vi "LED patterns.vi"() -> ()   [LabVIEW 2023]
uses:
  ctrl defs/ctrl number of LEDs.ctl
  ctrl defs/ctrl LED PATTERN DEFS.ctl
  ctrl defs/ctrl LED PATTERN SHAPES.ctl
  <vilib>/Rock Robotics/WPI/ThirdParty/JAS_Junk/TrajLib/MathUtil_Clamp.vi
  <vilib>/Rock Robotics/WPI/ThirdParty/JAS_Junk/TrajLib/Util_GetTime.vi
  <vilib>/Rock Robotics/WPI/ThirdParty/JAS_Junk/TrajLib/VI/Util_GetTime_U32.vi
  Global odometry.vi
  <vilib>/Rock Robotics/SystemInterfaces/Utilities/FPGA_UtilitiesRead LocalTime.vi
  <vilib>/Rock Robotics/WPI/ThirdParty/JAS_Junk/TrajLib/VI/Util_GetTime_U64.vi
  Global INIT.vi
  <vilib>/Rock Robotics/WPI/ThirdParty/JAS_Junk/TrajLib/Trajectory_Library.lvlib
panel:
  out "PATTERN SELECTED":T1=enum."WHITE, PULSE"
  out "decimated array 2":dbl[](array[numeric])
  out "decimated array":dbl[](array[numeric])
  out "Numeric":dbl
  out "FIBONACCI array":dbl[](array[numeric])
  out "HEARTBEAT":i32=54716
  in  "Dk BLUE":u32(colorbox)=721055
  in  "FUSCIA":u32(colorbox)=13107455
  in  "VIOLET":u32(colorbox)=5249480
  in  "PINK":u32(colorbox)=16070299
  in  "YELLOW":u32(colorbox)=16776960
  in  "ORANGE":u32(colorbox)=15156737
  in  "GREEN":u32(colorbox)=65280
  in  "Color2":u32(colorbox)=14535680 caption="Team\nColor\nSECOND"
  in  "Color1":u32(colorbox)=20922 caption="Team\nColor\nMAIN"
  out "SINE 0-1":dbl=0.9567727288213003
  out "SCAN rotation":dbl=47.83863644106501
  out "array DK BLUE":u32[](array[numeric])=[721055, 721055, 721055, 721055, 721055, 721055, 721055, 721055, 721055, 721055, 721055, 721055, 721055, 721055, 721055, 721055, 721055, 721055, 721055, 721055, 721055, 721055, 721055, 721055, 721055, 721055, 721055, 721055, 721055, 721055, 721055, 721055, 721055, 721055, 721055, 721055, 721055, 721055, 721055, 721055, 721055, 721055, 721055, 721055, 721055, 721055, 721055, 721055, 721055, 721055, 721055, 721055, 721055, 721055, 721055, 721055, 721055, 721055, 721055, 721055]
  in  "TESTING?":bool
  out "error out":errorcluster
  in  "error in (no error)":errorcluster
  out "LED WRITE 3":u32[](array[colorbox])
  out "LED WRITE 2":u32[](array[colorbox])=[0, 0, 0, 0, 0, 0, 0, 0, 20922, 20922, 20922, 20922, 20922, 20922, 20922, 20922, 20922, 20922, 0, 0]
  out "LED WRITE":u32[](array[colorbox])=[0, 0, 14535680, 14535680, 14535680, 14535680, 14535680, 14535680, 14535680, 14535680, 14535680, 14535680, 0, 0, 0, 0, 0, 0, 0, 0, 0, 0, 0, 0, 0, 0, 0, 0, 0, 0, 0, 0, 0, 0, 0, 0, 0, 0, 0, 0, 0, 0, 0, 0, 0, 0, 0, 0, 20922, 20922, 20922, 20922, 20922, 20922, 20922, 20922, 20922, 20922, 0, 0]
  in  "LOOP - BLINK (ms)":dbl=25.0
  in  "LOOP - BUMPER (ms)":dbl=10.0
  in  "LOOP - SCAN (ms)":dbl=10.0
  in  "LOOP - PULSE (ms)":dbl=10.0
  in  "LOOP - WAVE (ms)":dbl=10.0
  out "AdjustedWaitTime_MS":u32
  in  "DesiredLoopTime_MS":dbl=25.0 format="%#_13g"
  out "array AQUA":u32[](array[numeric])=[61414, 61414, 61414, 61414, 61414, 61414, 61414, 61414, 61414, 61414, 61414, 61414, 61414, 61414, 61414, 61414, 61414, 61414, 61414, 61414, 61414, 61414, 61414, 61414, 61414, 61414, 61414, 61414, 61414, 61414, 61414, 61414, 61414, 61414, 61414, 61414, 61414, 61414, 61414, 61414, 61414, 61414, 61414, 61414, 61414, 61414, 61414, 61414, 61414, 61414, 61414, 61414, 61414, 61414, 61414, 61414, 61414, 61414, 61414, 61414]
  out "array PINK":u32[](array[numeric])=[16711808, 16711808, 16711808, 16711808, 16711808, 16711808, 16711808, 16711808, 16711808, 16711808, 16711808, 16711808, 16711808, 16711808, 16711808, 16711808, 16711808, 16711808, 16711808, 16711808, 16711808, 16711808, 16711808, 16711808, 16711808, 16711808, 16711808, 16711808, 16711808, 16711808, 16711808, 16711808, 16711808, 16711808, 16711808, 16711808, 16711808, 16711808, 16711808, 16711808, 16711808, 16711808, 16711808, 16711808, 16711808, 16711808, 16711808, 16711808, 16711808, 16711808, 16711808, 16711808, 16711808, 16711808, 16711808, 16711808, 16711808, 16711808, 16711808, 16711808]
  out "array YELLOW":u32[](array[numeric])=[16449369, 16449369, 16449369, 16449369, 16449369, 16449369, 16449369, 16449369, 16449369, 16449369, 16449369, 16449369, 16449369, 16449369, 16449369, 16449369, 16449369, 16449369, 16449369, 16449369, 16449369, 16449369, 16449369, 16449369, 16449369, 16449369, 16449369, 16449369, 16449369, 16449369, 16449369, 16449369, 16449369, 16449369, 16449369, 16449369, 16449369, 16449369, 16449369, 16449369, 16449369, 16449369, 16449369, 16449369, 16449369, 16449369, 16449369, 16449369, 16449369, 16449369, 16449369, 16449369, 16449369, 16449369, 16449369, 16449369, 16449369, 16449369, 16449369, 16449369]
  out "SINE WAVE 1/2":u32[](array[numeric])=[0, 3, 11, 24, 42, 64, 88, 114, 141, 167, 191, 213, 231, 244, 252, 255, 252, 244, 231, 213, 191, 167, 141, 114, 88, 64, 42, 24, 11, 3, 0, 3, 11, 24, 42, 64, 88, 114, 141, 167, 191, 213, 231, 244, 252, 255, 252, 244, 231, 213, 191, 167, 141, 114, 88, 64, 42, 24, 11, 3]
  out "SINE WAVE":u32[](array[numeric])=[0, 1, 3, 6, 11, 17, 24, 33, 42, 53, 64, 76, 88, 101, 114, 128, 141, 154, 167, 179, 191, 202, 213, 222, 231, 238, 244, 249, 252, 254, 255, 254, 252, 249, 244, 238, 231, 222, 213, 202, 191, 179, 167, 154, 141, 128, 114, 101, 88, 76, 64, 53, 42, 33, 24, 17, 11, 6, 3, 1]
  out "REVERSE BUMP":i8=49
  out "FORWARD INDEX":i32=29
  out "REVERSE INDEX":i32=30
  in  "slider length":i8=10
  out "array EMPTY":u32[](array[numeric])=[1073741824, 1073741824, 1073741824, 1073741824, 1073741824, 1073741824, 1073741824, 1073741824, 1073741824, 1073741824, 1073741824, 1073741824, 1073741824, 1073741824, 1073741824, 1073741824, 1073741824, 1073741824, 1073741824, 1073741824, 1073741824, 1073741824, 1073741824, 1073741824, 1073741824, 1073741824, 1073741824, 1073741824, 1073741824, 1073741824, 1073741824, 1073741824, 1073741824, 1073741824, 1073741824, 1073741824, 1073741824, 1073741824, 1073741824, 1073741824, 1073741824, 1073741824, 1073741824, 1073741824, 1073741824, 1073741824, 1073741824, 1073741824, 1073741824, 1073741824, 1073741824, 1073741824, 1073741824, 1073741824, 1073741824, 1073741824, 1073741824, 1073741824, 1073741824, 1073741824]
  out "SLIDER BLACK":u32[](array[colorbox])
  out "array BLUE":u32[](array[numeric])=[220, 220, 220, 220, 220, 220, 220, 220, 220, 220, 220, 220, 220, 220, 220, 220, 220, 220, 220, 220, 220, 220, 220, 220, 220, 220, 220, 220, 220, 220, 220, 220, 220, 220, 220, 220, 220, 220, 220, 220, 220, 220, 220, 220, 220, 220, 220, 220, 220, 220, 220, 220, 220, 220, 220, 220, 220, 220, 220, 220]
  out "array FUSCIA":u32[](array[numeric])=[16711934, 16711934, 16711934, 16711934, 16711934, 16711934, 16711934, 16711934, 16711934, 16711934, 16711934, 16711934, 16711934, 16711934, 16711934, 16711934, 16711934, 16711934, 16711934, 16711934, 16711934, 16711934, 16711934, 16711934, 16711934, 16711934, 16711934, 16711934, 16711934, 16711934, 16711934, 16711934, 16711934, 16711934, 16711934, 16711934, 16711934, 16711934, 16711934, 16711934, 16711934, 16711934, 16711934, 16711934, 16711934, 16711934, 16711934, 16711934, 16711934, 16711934, 16711934, 16711934, 16711934, 16711934, 16711934, 16711934, 16711934, 16711934, 16711934, 16711934]
  out "array ORANGE":u32[](array[numeric])=[16748288, 16748288, 16748288, 16748288, 16748288, 16748288, 16748288, 16748288, 16748288, 16748288, 16748288, 16748288, 16748288, 16748288, 16748288, 16748288, 16748288, 16748288, 16748288, 16748288, 16748288, 16748288, 16748288, 16748288, 16748288, 16748288, 16748288, 16748288, 16748288, 16748288, 16748288, 16748288, 16748288, 16748288, 16748288, 16748288, 16748288, 16748288, 16748288, 16748288, 16748288, 16748288, 16748288, 16748288, 16748288, 16748288, 16748288, 16748288, 16748288, 16748288, 16748288, 16748288, 16748288, 16748288, 16748288, 16748288, 16748288, 16748288, 16748288, 16748288]
  out "array COLOR1":u32[](array[numeric])=[191, 191, 191, 191, 191, 191, 191, 191, 191, 191, 191, 191, 191, 191, 191, 191, 191, 191, 191, 191, 191, 191, 191, 191, 191, 191, 191, 191, 191, 191, 191, 191, 191, 191, 191, 191, 191, 191, 191, 191, 191, 191, 191, 191, 191, 191, 191, 191, 191, 191, 191, 191, 191, 191, 191, 191, 191, 191, 191, 191]
  out "array COLOR2":u32[](array[numeric])=[14794496, 14794496, 14794496, 14794496, 14794496, 14794496, 14794496, 14794496, 14794496, 14794496, 14794496, 14794496, 14794496, 14794496, 14794496, 14794496, 14794496, 14794496, 14794496, 14794496, 14794496, 14794496, 14794496, 14794496, 14794496, 14794496, 14794496, 14794496, 14794496, 14794496, 14794496, 14794496, 14794496, 14794496, 14794496, 14794496, 14794496, 14794496, 14794496, 14794496, 14794496, 14794496, 14794496, 14794496, 14794496, 14794496, 14794496, 14794496, 14794496, 14794496, 14794496, 14794496, 14794496, 14794496, 14794496, 14794496, 14794496, 14794496, 14794496, 14794496]
  out "array RED":u32[](array[numeric])=[16711680, 16711680, 16711680, 16711680, 16711680, 16711680, 16711680, 16711680, 16711680, 16711680, 16711680, 16711680, 16711680, 16711680, 16711680, 16711680, 16711680, 16711680, 16711680, 16711680, 16711680, 16711680, 16711680, 16711680, 16711680, 16711680, 16711680, 16711680, 16711680, 16711680, 16711680, 16711680, 16711680, 16711680, 16711680, 16711680, 16711680, 16711680, 16711680, 16711680, 16711680, 16711680, 16711680, 16711680, 16711680, 16711680, 16711680, 16711680, 16711680, 16711680, 16711680, 16711680, 16711680, 16711680, 16711680, 16711680, 16711680, 16711680, 16711680, 16711680]
  out "array GREEN":u32[](array[numeric])=[65280, 65280, 65280, 65280, 65280, 65280, 65280, 65280, 65280, 65280, 65280, 65280, 65280, 65280, 65280, 65280, 65280, 65280, 65280, 65280, 65280, 65280, 65280, 65280, 65280, 65280, 65280, 65280, 65280, 65280, 65280, 65280, 65280, 65280, 65280, 65280, 65280, 65280, 65280, 65280, 65280, 65280, 65280, 65280, 65280, 65280, 65280, 65280, 65280, 65280, 65280, 65280, 65280, 65280, 65280, 65280, 65280, 65280, 65280, 65280]
  out "array WHITE":u32[](array[numeric])=[16448250, 16448250, 16448250, 16448250, 16448250, 16448250, 16448250, 16448250, 16448250, 16448250, 16448250, 16448250, 16448250, 16448250, 16448250, 16448250, 16448250, 16448250, 16448250, 16448250, 16448250, 16448250, 16448250, 16448250, 16448250, 16448250, 16448250, 16448250, 16448250, 16448250, 16448250, 16448250, 16448250, 16448250, 16448250, 16448250, 16448250, 16448250, 16448250, 16448250, 16448250, 16448250, 16448250, 16448250, 16448250, 16448250, 16448250, 16448250, 16448250, 16448250, 16448250, 16448250, 16448250, 16448250, 16448250, 16448250, 16448250, 16448250, 16448250, 16448250]
  out "array BLACK":u32[](array[numeric])
  out "array VIOLET":u32[](array[numeric])=[11152127, 11152127, 11152127, 11152127, 11152127, 11152127, 11152127, 11152127, 11152127, 11152127, 11152127, 11152127, 11152127, 11152127, 11152127, 11152127, 11152127, 11152127, 11152127, 11152127, 11152127, 11152127, 11152127, 11152127, 11152127, 11152127, 11152127, 11152127, 11152127, 11152127, 11152127, 11152127, 11152127, 11152127, 11152127, 11152127, 11152127, 11152127, 11152127, 11152127, 11152127, 11152127, 11152127, 11152127, 11152127, 11152127, 11152127, 11152127, 11152127, 11152127, 11152127, 11152127, 11152127, 11152127, 11152127, 11152127, 11152127, 11152127, 11152127, 11152127]
  out "SLIDER WHITE":u32[](array[colorbox])=[16448250, 16448250, 16448250, 16448250, 16448250, 16448250, 16448250, 16448250, 16448250, 16448250]
  in  "TEST - PATTERN SELECT":T1=enum."CROSSING, COLORS 1&2"
  out "#LEDs":T2=60
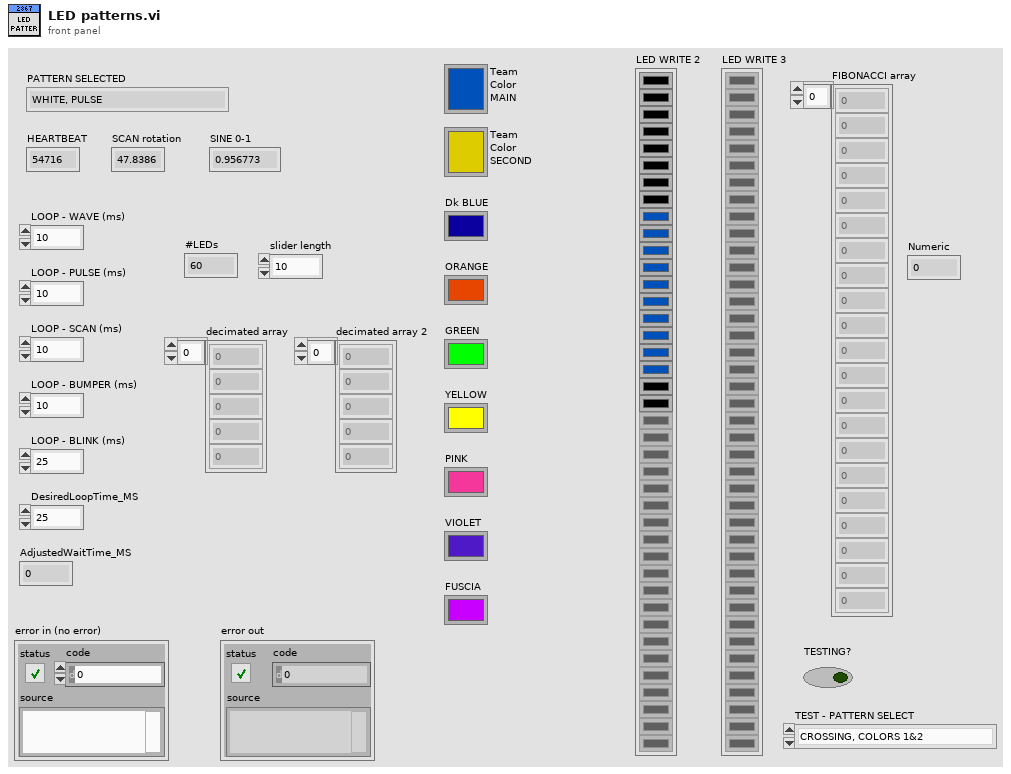
[diagram p1: front panel]
types:
  T1 = typedef "ctrl LED PATTERN DEFS.ctl" = enum16{"default", "RED, SOLID", "RED, BUMPER", "RED, BLINK", "RED, WAVE", "RED, SCAN", "RED, PULSE", "BLUE, SOLID", "BLUE, BUMPER", "BLUE, BLINK", "BLUE, WAVE", "BLUE, SCAN", "BLUE, PULSE", "GREEN, SOLID", "GREEN, BUMPER", "GREEN, BLINK", "GREEN, WAVE", "GREEN, SCAN", "GREEN, PULSE", "WHITE, WAVE", "WHITE, PULSE", "COLOR 1 scan white", "COLOR 1 scan COLOR 2", "COLOR 1 bumper white", "COLOR 1 bumper COLOR 2", "PINK, SOLID", "PINK, BLINK", "VIOLET, SOLID", "VIOLET, BLINK", "ORANGE, SOLID", "ORANGE, BLINK", "YELLOW, SOLID", "YELLOW, BLINK", "FUSCIA, SOLID", "FUSCIA, BLINK", "AQUA, SOLID", "AQUA, BLINK", "AQUA, BUMPER", "AQUA, SCAN", "FUSCIA, BUMPER", "FUSCIA, SCAN", "ORANGE, BUMPER", "ORANGE, SCAN", "VIOLET, BUMPER", "VIOLET, SCAN", "YELLOW, BUMPER", "YELLOW, SCAN", "PINK, BUMPER", "PINK, SCAN", "CROSSING, RED & BLUE", "CROSSING, COLORS 1&2", "TEST", "RAINBOW", "RED, EXPAND", "BLUE, EXPAND", "GREEN, EXPAND", "RED, EX-CON", "BLUE, EX-CON", "GREEN, EX-CON", "EMERGENCY STOP", "LOW BATTERY"}
  T2 = typedef "ctrl number of LEDs.ctl" = u16
  T3 = typedef "ctrl LED PATTERN SHAPES.ctl" = enum16{"SOLID", "BUMPER", "SCAN", "WAVE", "EXPAND", "EX-CON", "CROSS", "BLINK", "PULSE", "SCAN FAST", "BUMPER FAST", "FIBONACCI"}
  T4 = typedef "ctrl LED init.ctl" = cluster{"PWM Channel":T5, "refnum name":string, "#LEDS":T2, "initial output":dbl, "stack name":string, "Installed?":bool, "pattern":T6}
  T5 = typedef "FPGA_DIOPWMChannel.ctl" = enum8{"PWM 0", "PWM 1", "PWM 2", "PWM 3", "PWM 4", "PWM 5", "PWM 6", "PWM 7", "PWM 8", "PWM 9", "PWM MXP 0", "PWM MXP 1", "PWM MXP 2", "PWM MXP 3", "PWM MXP 4", "PWM MXP 5", "PWM MXP 6", "PWM MXP 7", "PWM MXP 8", "PWM MXP 9", "Invalid"}
  T6 = typedef "ctrl LED PATTERNS.ctl" = u16
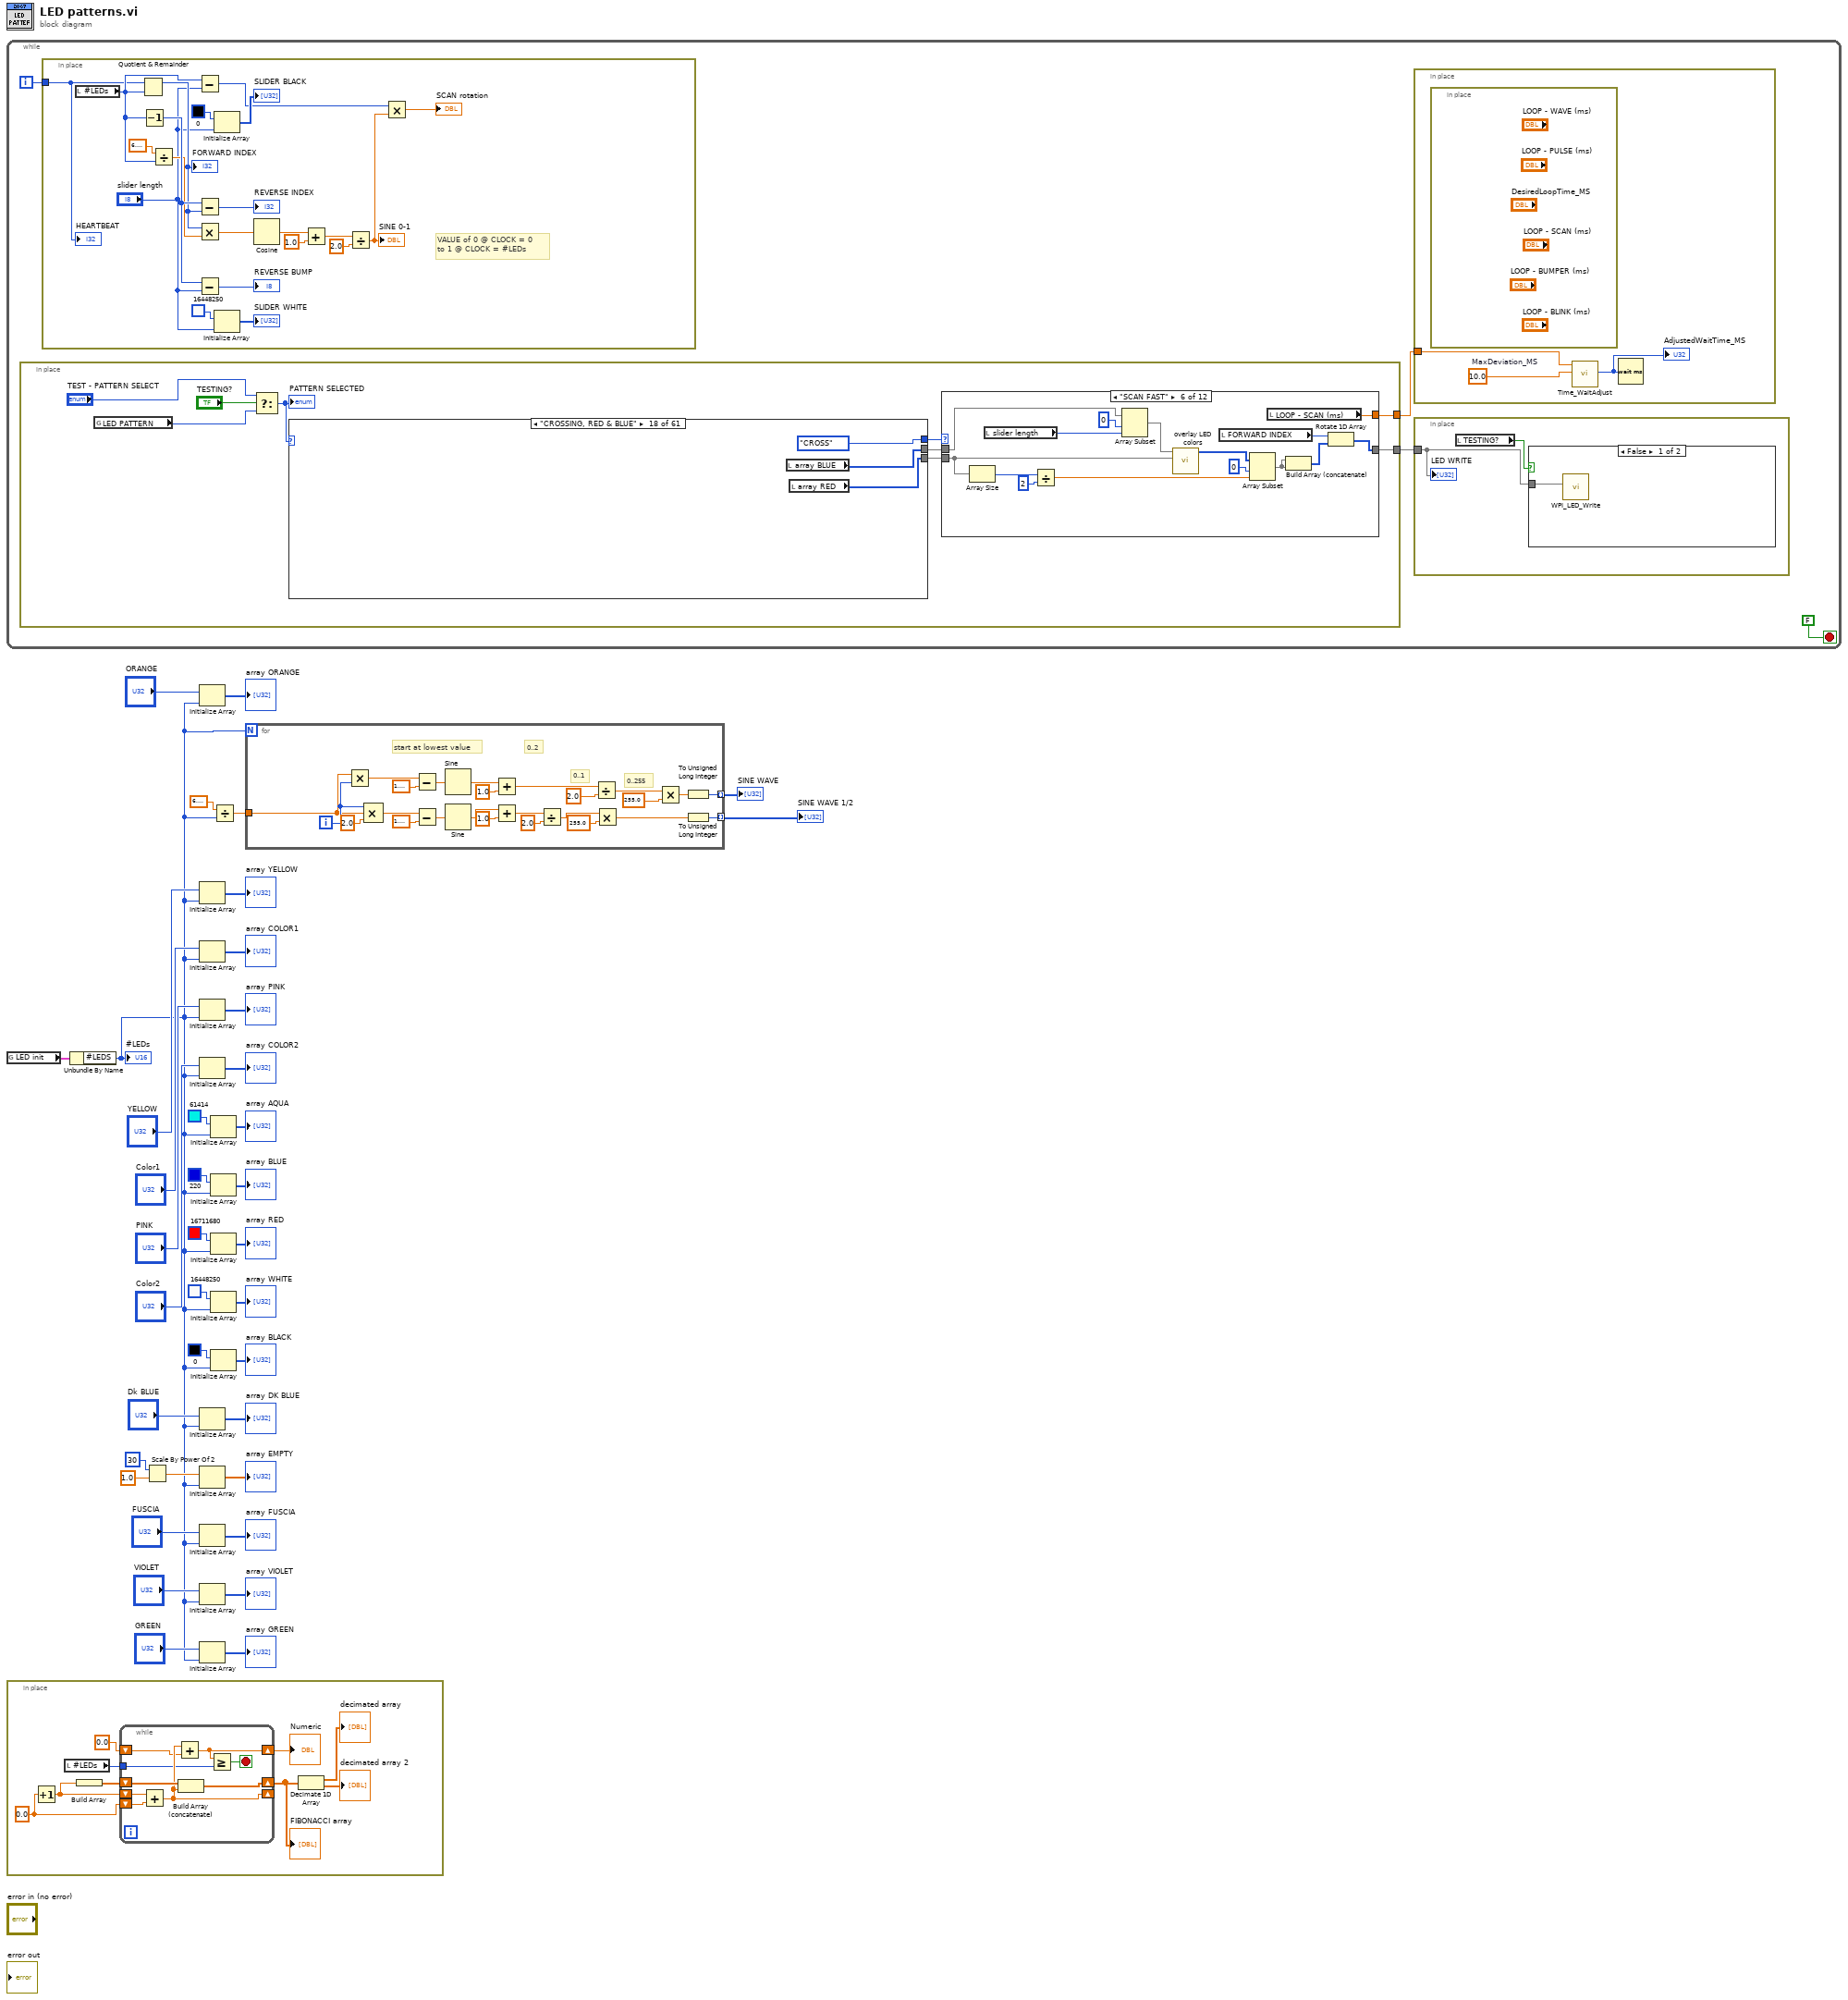
[diagram p0: block diagram]
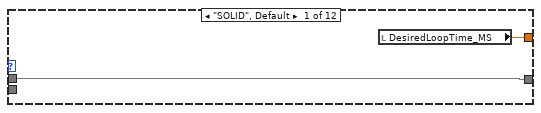
[diagram p2: hidden frame]
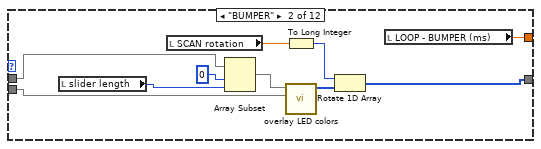
[diagram p3: hidden frame]
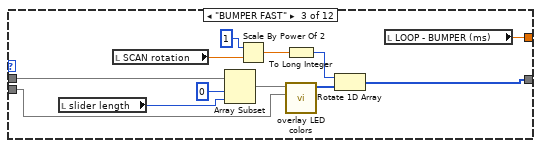
[diagram p4: hidden frame]
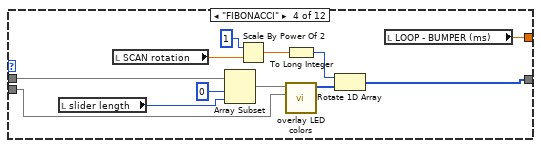
[diagram p5: hidden frame]
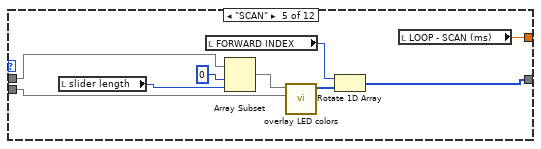
[diagram p6: hidden frame]
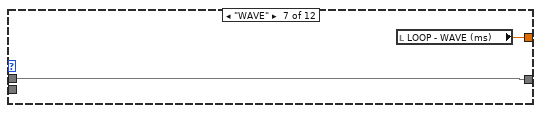
[diagram p7: hidden frame]
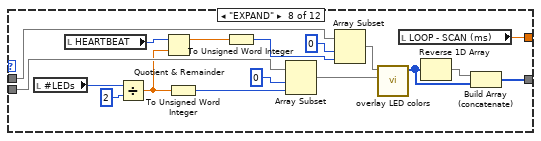
[diagram p8: hidden frame]
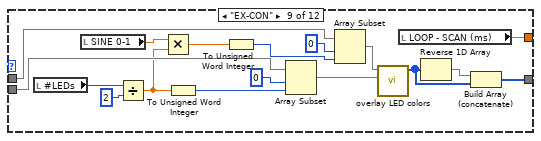
[diagram p9: hidden frame]
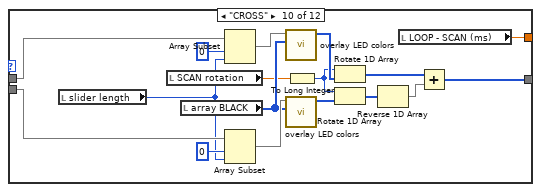
[diagram p10: hidden frame]
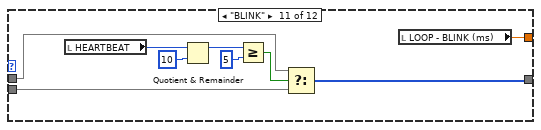
[diagram p11: hidden frame]
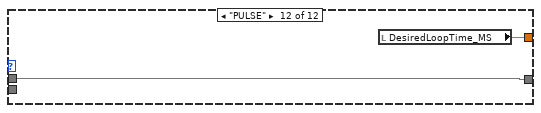
[diagram p12: hidden frame]
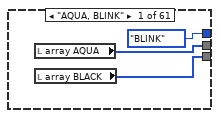
[diagram p13: hidden frame]
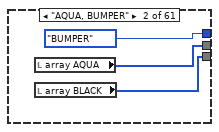
[diagram p14: hidden frame]
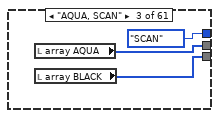
[diagram p15: hidden frame]
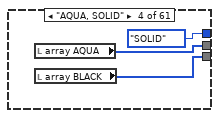
[diagram p16: hidden frame]
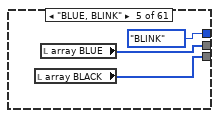
[diagram p17: hidden frame]
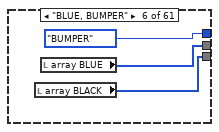
[diagram p18: hidden frame]
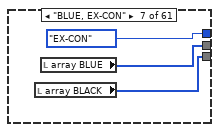
[diagram p19: hidden frame]
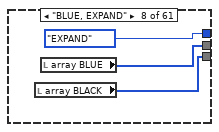
[diagram p20: hidden frame]
diagram:
  n1 = while {
    i -> [w42]
    stop <- FALSE stop-if-true
    n2 = in-place {
      in-place-border: [w50] -> w41
      in-place-border: [w48] -> w40
      n3 = global read "Global odometry.vi" "LED PATTERN"() -> (w43:T1)
      n4 = Select(t="TEST - PATTERN SELECT", s="TESTING?", f=w43) -> (s? t:f=w46:T1)
      "PATTERN SELECTED" <- w46
      n5 = case shown="\"CROSSING, RED & BLUE\"" w46 {
        tunnel: [w178 w181 w184 w187 w190 w193 w196 w199 w206 w209 w211 w218 w221 w223 w226 w240 w246 w249 w252 w256 w259 w262 w265 w268 w271 w274 w277 w284 w287 w290 w297 w300 w303 w306 w309 w311 w315 w318 w321 w323 w335 w337 w341 w344 w351 w354 w356 w363 w366 w369 w372 w377 w390 w410 w412 w414 w425 w437 w440 w443 w446] -> w51
        tunnel: [w177 w180 w183 w186 w189 w192 w195 w198 w201 w208 w211 w213 w220 w224 w226 w240 w247 w250 w252 w255 w258 w261 w264 w267 w270 w273 w276 w279 w286 w289 w292 w299 w302 w305 w308 w310 w314 w317 w320 w323 w334 w338 w340 w343 w346 w353 w356 w358 w365 w368 w371 w377 w390 w409 w411 w414 w425 w436 w439 w442 w445] -> w49
        tunnel: [ctrl_LED_PATTERN_SHAPES."BLINK" ctrl_LED_PATTERN_SHAPES."BUMPER" ctrl_LED_PATTERN_SHAPES."SCAN" ctrl_LED_PATTERN_SHAPES."SOLID" ctrl_LED_PATTERN_SHAPES."BLINK" ctrl_LED_PATTERN_SHAPES."BUMPER" ctrl_LED_PATTERN_SHAPES."EX-CON" ctrl_LED_PATTERN_SHAPES."EXPAND" ctrl_LED_PATTERN_SHAPES."PULSE" ctrl_LED_PATTERN_SHAPES."SCAN" ctrl_LED_PATTERN_SHAPES."SOLID" ctrl_LED_PATTERN_SHAPES."WAVE" ctrl_LED_PATTERN_SHAPES."BUMPER" ctrl_LED_PATTERN_SHAPES."BUMPER" ctrl_LED_PATTERN_SHAPES."SOLID" ctrl_LED_PATTERN_SHAPES."SCAN" ctrl_LED_PATTERN_SHAPES."CROSS" ctrl_LED_PATTERN_SHAPES."CROSS" ctrl_LED_PATTERN_SHAPES."SOLID" ctrl_LED_PATTERN_SHAPES."BLINK" ctrl_LED_PATTERN_SHAPES."BUMPER" ctrl_LED_PATTERN_SHAPES."SCAN" ctrl_LED_PATTERN_SHAPES."SOLID" ctrl_LED_PATTERN_SHAPES."BLINK" ctrl_LED_PATTERN_SHAPES."BUMPER" ctrl_LED_PATTERN_SHAPES."EX-CON" ctrl_LED_PATTERN_SHAPES."EXPAND" ctrl_LED_PATTERN_SHAPES."PULSE" ctrl_LED_PATTERN_SHAPES."SCAN" ctrl_LED_PATTERN_SHAPES."SOLID" ctrl_LED_PATTERN_SHAPES."WAVE" ctrl_LED_PATTERN_SHAPES."BLINK" ctrl_LED_PATTERN_SHAPES."BUMPER" ctrl_LED_PATTERN_SHAPES."SCAN FAST" ctrl_LED_PATTERN_SHAPES."SOLID" ctrl_LED_PATTERN_SHAPES."BLINK" ctrl_LED_PATTERN_SHAPES."BUMPER" ctrl_LED_PATTERN_SHAPES."SCAN" ctrl_LED_PATTERN_SHAPES."SOLID" ctrl_LED_PATTERN_SHAPES."SOLID" ctrl_LED_PATTERN_SHAPES."BLINK" ctrl_LED_PATTERN_SHAPES."BUMPER" ctrl_LED_PATTERN_SHAPES."EX-CON" ctrl_LED_PATTERN_SHAPES."EXPAND" ctrl_LED_PATTERN_SHAPES."PULSE" ctrl_LED_PATTERN_SHAPES."SCAN FAST" ctrl_LED_PATTERN_SHAPES."SOLID" ctrl_LED_PATTERN_SHAPES."WAVE" ctrl_LED_PATTERN_SHAPES."SCAN" ctrl_LED_PATTERN_SHAPES."BLINK" ctrl_LED_PATTERN_SHAPES."BUMPER" ctrl_LED_PATTERN_SHAPES."SCAN" ctrl_LED_PATTERN_SHAPES."SCAN" ctrl_LED_PATTERN_SHAPES."SCAN" ctrl_LED_PATTERN_SHAPES."SOLID" ctrl_LED_PATTERN_SHAPES."SOLID" ctrl_LED_PATTERN_SHAPES."SOLID" ctrl_LED_PATTERN_SHAPES."BLINK" ctrl_LED_PATTERN_SHAPES."BUMPER" ctrl_LED_PATTERN_SHAPES."SCAN" ctrl_LED_PATTERN_SHAPES."SOLID"] -> w47
        frame "AQUA, BLINK" {
          n6 = local read "array AQUA"() -> (w178:u32[])
          n7 = local read "array BLACK"() -> (w177:u32[])
        }
        frame "AQUA, BUMPER" {
          n8 = local read "array AQUA"() -> (w181:u32[])
          n9 = local read "array BLACK"() -> (w180:u32[])
        }
        frame "AQUA, SCAN" {
          n10 = local read "array AQUA"() -> (w184:u32[])
          n11 = local read "array BLACK"() -> (w183:u32[])
        }
        frame "AQUA, SOLID" {
          n12 = local read "array AQUA"() -> (w187:u32[])
          n13 = local read "array BLACK"() -> (w186:u32[])
        }
        frame "BLUE, BLINK" {
          n14 = local read "array BLACK"() -> (w189:u32[])
          n15 = local read "array BLUE"() -> (w190:u32[])
        }
        frame "BLUE, BUMPER" {
          n16 = local read "array BLACK"() -> (w192:u32[])
          n17 = local read "array BLUE"() -> (w193:u32[])
        }
        frame "BLUE, EX-CON" {
          n18 = local read "array BLACK"() -> (w195:u32[])
          n19 = local read "array BLUE"() -> (w196:u32[])
        }
        frame "BLUE, EXPAND" {
          n20 = local read "array BLACK"() -> (w198:u32[])
          n21 = local read "array BLUE"() -> (w199:u32[])
        }
        frame "BLUE, PULSE" {
          n22 = local read "SINE WAVE 1/2"() -> (w205:u32[])
          n23 = local read "FORWARD INDEX"() -> (w204:i32)
          n24 = Logical Shift(y=i16 0, x=w205) -> (x << y=w203:u32[])
          n25 = local read "array BLACK"() -> (w201:u32[])
          n26 = Rotate 1D Array(1:w203, 2:w204) -> (0:w206:u32[])
        }
        frame "BLUE, SCAN" {
          n27 = local read "array BLACK"() -> (w208:u32[])
          n28 = local read "array BLUE"() -> (w209:u32[])
        }
        frame "BLUE, SOLID" {
          n29 = local read "array BLUE"() -> (w211:u32[])
        }
        frame "BLUE, WAVE" {
          n30 = local read "SINE WAVE"() -> (w217:u32[])
          n31 = local read "FORWARD INDEX"() -> (w216:i32)
          n32 = Logical Shift(y=i16 0, x=w217) -> (x << y=w215:u32[])
          n33 = local read "array BLACK"() -> (w213:u32[])
          n34 = Rotate 1D Array(1:w215, 2:w216) -> (0:w218:u32[])
        }
        frame "COLOR 1 bumper COLOR 2" {
          n35 = local read "array COLOR2"() -> (w221:u32[])
          n36 = local read "array COLOR1"() -> (w220:u32[])
        }
        frame "COLOR 1 bumper white" {
          n37 = local read "array COLOR1"() -> (w224:u32[])
          n38 = local read "array WHITE"() -> (w223:u32[])
        }
        frame "COLOR 1 scan COLOR 2" {
          n39 = local read "Color2"() -> (w236:u32)
          n40 = Initialize Array(w236, 10 ("dimension size")) -> (w235:u32[])
          n41 = local read "array COLOR1"() -> (w238:u32[])
          n42 = local read "#LEDs"() -> (w231:T2)
          n43 = call "overlay LED colors.vi"("BASE ARRAY"=w238, "OVERLAY"=w235) -> ("BLENDED ARRAY"=w233:u32[])  [unwired: 9 in]
          n44 = Quotient & Remainder(x=w231, y=i8 3) -> (floor(x/y)=w229:T2)  [unwired: 1 out]
          n45 = local read "FORWARD INDEX"() -> (w237:i32)
          n46 = Array Subset(array=w233, index=0, length=w229) -> (w228:u32[])
          n47 = Build Array (concatenate)(w228, w228, w228) -> (w227:u32[])
          n48 = Rotate 1D Array(1:w227, 2:w237) -> (0:w226:u32[])
        }
        frame "COLOR 1 scan white" {
          n49 = local read "SLIDER WHITE"() -> (w244:u32[])
          n50 = local read "array COLOR1"() -> (w243:u32[])
          n51 = local read "FORWARD INDEX"() -> (w241:i32)
          n52 = call "overlay LED colors.vi"("BASE ARRAY"=w243, "OVERLAY"=w244) -> ("BLENDED ARRAY"=w242:u32[])  [unwired: 9 in]
          n53 = Rotate 1D Array(1:w242, 2:w241) -> (0:w240:u32[])
        }
        frame "CROSSING, COLORS 1&2" {
          n54 = local read "array COLOR1"() -> (w246:u32[])
          n55 = local read "array COLOR2"() -> (w247:u32[])
        }
        frame "CROSSING, RED & BLUE" {
          n56 = local read "array BLUE"() -> (w249:u32[])
          n57 = local read "array RED"() -> (w250:u32[])
        }
        frame "default", Default {
          n58 = local write "TEST - PATTERN SELECT"(ctrl_LED_PATTERN_DEFS."COLOR 1 bumper COLOR 2" ("PATTERN SELECT")) -> ()
          n59 = local read "array BLACK"() -> (w252:u32[])
        }
        frame "FUSCIA, BLINK" {
          n60 = local read "array FUSCIA"() -> (w256:u32[])
          n61 = local read "array BLACK"() -> (w255:u32[])
        }
        frame "FUSCIA, BUMPER" {
          n62 = local read "array FUSCIA"() -> (w259:u32[])
          n63 = local read "array BLACK"() -> (w258:u32[])
        }
        frame "FUSCIA, SCAN" {
          n64 = local read "array FUSCIA"() -> (w262:u32[])
          n65 = local read "array BLACK"() -> (w261:u32[])
        }
        frame "FUSCIA, SOLID" {
          n66 = local read "array FUSCIA"() -> (w265:u32[])
          n67 = local read "array BLACK"() -> (w264:u32[])
        }
        frame "GREEN, BLINK" {
          n68 = local read "array GREEN"() -> (w268:u32[])
          n69 = local read "array BLACK"() -> (w267:u32[])
        }
        frame "GREEN, BUMPER" {
          n70 = local read "array GREEN"() -> (w271:u32[])
          n71 = local read "array BLACK"() -> (w270:u32[])
        }
        frame "GREEN, EX-CON" {
          n72 = local read "array GREEN"() -> (w274:u32[])
          n73 = local read "array BLACK"() -> (w273:u32[])
        }
        frame "GREEN, EXPAND" {
          n74 = local read "array GREEN"() -> (w277:u32[])
          n75 = local read "array BLACK"() -> (w276:u32[])
        }
        frame "GREEN, PULSE" {
          n76 = local read "SINE WAVE 1/2"() -> (w283:u32[])
          n77 = local read "FORWARD INDEX"() -> (w282:i32)
          n78 = Logical Shift(y=i16 8, x=w283) -> (x << y=w281:u32[])
          n79 = local read "array BLACK"() -> (w279:u32[])
          n80 = Rotate 1D Array(1:w281, 2:w282) -> (0:w284:u32[])
        }
        frame "GREEN, SCAN" {
          n81 = local read "array GREEN"() -> (w287:u32[])
          n82 = local read "array BLACK"() -> (w286:u32[])
        }
        frame "GREEN, SOLID" {
          n83 = local read "array GREEN"() -> (w290:u32[])
          n84 = local read "array BLACK"() -> (w289:u32[])
        }
        frame "GREEN, WAVE" {
          n85 = local read "SINE WAVE"() -> (w296:u32[])
          n86 = local read "FORWARD INDEX"() -> (w295:i32)
          n87 = Logical Shift(y=i16 8, x=w296) -> (x << y=w294:u32[])
          n88 = local read "array BLACK"() -> (w292:u32[])
          n89 = Rotate 1D Array(1:w294, 2:w295) -> (0:w297:u32[])
        }
        frame "ORANGE, BLINK" {
          n90 = local read "array ORANGE"() -> (w300:u32[])
          n91 = local read "array BLACK"() -> (w299:u32[])
        }
        frame "ORANGE, BUMPER" {
          n92 = local read "array ORANGE"() -> (w303:u32[])
          n93 = local read "array BLACK"() -> (w302:u32[])
        }
        frame "ORANGE, SCAN" {
          n94 = local read "array ORANGE"() -> (w306:u32[])
          n95 = local read "array BLACK"() -> (w305:u32[])
        }
        frame "ORANGE, SOLID" {
          n96 = local read "array ORANGE"() -> (w309:u32[])
          n97 = local read "array BLACK"() -> (w308:u32[])
        }
        frame "PINK, BLINK" {
          n98 = local read "array BLACK"() -> (w310:u32[])
          n99 = local read "array PINK"() -> (w311:u32[])
        }
        frame "PINK, BUMPER" {
          n100 = local read "array BLACK"() -> (w314:u32[])
          n101 = local read "array PINK"() -> (w315:u32[])
        }
        frame "PINK, SCAN" {
          n102 = local read "array BLACK"() -> (w317:u32[])
          n103 = local read "array PINK"() -> (w318:u32[])
        }
        frame "PINK, SOLID" {
          n104 = local read "array BLACK"() -> (w320:u32[])
          n105 = local read "array PINK"() -> (w321:u32[])
        }
        frame "RAINBOW" {
          n106 = local read "SINE WAVE"() -> (w328:u32[])
          n107 = local read "FORWARD INDEX"() -> (w326:i32)
          n108 = Logical Shift(y=i16 0, x=w328) -> (x << y=w331:u32[])
          n109 = Logical Shift(y=i16 16, x=w328) -> (x << y=w327:u32[])
          n110 = Rotate 1D Array(1:w331, 2:w326) -> (0:w332:u32[])
          n111 = Rotate 1D Array(1:w327, 2:w326) -> (0:w325:u32[])
          n112 = Reverse 1D Array(array=w325) -> (reversed array=w324:u32[])
          n113 = Add(x=w332, y=w324) -> (x+y=w323:u32[])
        }
        frame "RED, BLINK" {
          n114 = local read "array BLACK"() -> (w334:u32[])
          n115 = local read "array RED"() -> (w335:u32[])
        }
        frame "RED, BUMPER" {
          n116 = local read "array BLACK"() -> (w338:u32[])
          n117 = local read "array RED"() -> (w337:u32[])
        }
        frame "RED, EX-CON" {
          n118 = local read "array BLACK"() -> (w340:u32[])
          n119 = local read "array RED"() -> (w341:u32[])
        }
        frame "RED, EXPAND" {
          n120 = local read "array BLACK"() -> (w343:u32[])
          n121 = local read "array RED"() -> (w344:u32[])
        }
        frame "RED, PULSE" {
          n122 = local read "SINE WAVE 1/2"() -> (w350:u32[])
          n123 = local read "FORWARD INDEX"() -> (w349:i32)
          n124 = Logical Shift(y=i16 16, x=w350) -> (x << y=w348:u32[])
          n125 = local read "array BLACK"() -> (w346:u32[])
          n126 = Rotate 1D Array(1:w348, 2:w349) -> (0:w351:u32[])
        }
        frame "RED, SCAN" {
          n127 = local read "array BLACK"() -> (w353:u32[])
          n128 = local read "array RED"() -> (w354:u32[])
        }
        frame "RED, SOLID" {
          n129 = local read "array RED"() -> (w356:u32[])
        }
        frame "RED, WAVE" {
          n130 = local read "SINE WAVE"() -> (w362:u32[])
          n131 = local read "FORWARD INDEX"() -> (w361:i32)
          n132 = Logical Shift(y=i16 16, x=w362) -> (x << y=w360:u32[])
          n133 = local read "array BLACK"() -> (w358:u32[])
          n134 = Rotate 1D Array(1:w360, 2:w361) -> (0:w363:u32[])
        }
        frame "TEST" {
          n135 = local read "array BLACK"() -> (w365:u32[])
          n136 = local read "array PINK"() -> (w366:u32[])
        }
        frame "VIOLET, BLINK" {
          n137 = local read "array VIOLET"() -> (w369:u32[])
          n138 = local read "array BLACK"() -> (w368:u32[])
        }
        frame "VIOLET, BUMPER" {
          n139 = local read "array VIOLET"() -> (w372:u32[])
          n140 = local read "array BLACK"() -> (w371:u32[])
        }
        frame "EMERGENCY STOP" {
          w382 = 0 ("index")
          n141 = local read "#LEDs"() -> (w385:T2)
          n142 = local read "array YELLOW"() -> (w383:u32[])
          n143 = local read "array RED"() -> (w375:u32[])
          n144 = Quotient & Remainder(x=w385, y=T2 8) -> (x-y*floor(x/y)=w373:T2, floor(x/y)=w381:T2)
          n145 = Array Subset(array=w375, index=w382, length=w381) -> (w380:u32[])
          n146 = Array Subset(array=w383, index=w382, length=w381) -> (w379:u32[])
          n147 = Array Subset(array=w375, index=0, length=w373) -> (w376:u32[])
          n148 = Build Array (concatenate)(w380, w379) -> (w378:u32[])
          n149 = Build Array (concatenate)(w378, w378, w378, w378, w376) -> (w377:u32[])
        }
        frame "LOW BATTERY" {
          w403 = 0 ("index")
          w401 = T2 3 ("y")
          n150 = local read "array YELLOW"() -> (w402:u32[])
          n151 = local read "array RED"() -> (w397:u32[])
          n152 = local read "#LEDs"() -> (w388:T2)
          n153 = Array Subset(array=w397, index=w403, length=w401) -> (w400:u32[])
          n154 = Array Subset(array=w402, index=w403, length=w401) -> (w399:u32[])
          n155 = Quotient & Remainder(x=w388, y=w401) -> (x-y*floor(x/y)=w395:T2, floor(x/y)=w398:T2)
          n156 = Build Array (concatenate)(w400, w399) -> (w391:u32[])
          n157 = for {
            N: w398 -> [_]
            tunnel: w391 -> [w406]
            shift-right: [w405] -> w394
            shift-left: w391 -> [w407]
            n158 = Build Array (concatenate)(w407, w406) -> (w405:u32[])
          }
          n159 = Array Subset(array=w397, index=0, length=w395) -> (w393:u32[])
          n160 = Build Array (concatenate)(w394, w393) -> (w392:u32[])
          n161 = Decrement(x=w388) -> (x-1=w387:T2)
          n162 = Array Subset(array=w392, index=0, length=w387) -> (w390:u32[])
        }
        frame "VIOLET, SCAN" {
          n163 = local read "array VIOLET"() -> (w410:u32[])
          n164 = local read "array BLACK"() -> (w409:u32[])
        }
        frame "VIOLET, SOLID" {
          n165 = local read "array VIOLET"() -> (w412:u32[])
          n166 = local read "array BLACK"() -> (w411:u32[])
        }
        frame "WHITE, PULSE" {
          n167 = local read "SINE WAVE 1/2"() -> (w416:u32[])
          n168 = local read "FORWARD INDEX"() -> (w424:i32)
          n169 = Logical Shift(y=i16 0, x=w416) -> (x << y=w419:u32[])
          n170 = Logical Shift(y=i16 8, x=w416) -> (x << y=w418:u32[])
          n171 = Logical Shift(y=i16 16, x=w416) -> (x << y=w417:u32[])
          n172 = Compound Arithmetic op=ADD(w419, w418, w417) -> (w420:u32[])
          n173 = Rotate 1D Array(1:w420, 2:w424) -> (0:w414:u32[])
        }
        frame "WHITE, WAVE" {
          n174 = local read "SINE WAVE"() -> (w427:u32[])
          n175 = local read "FORWARD INDEX"() -> (w435:i32)
          n176 = Logical Shift(y=i16 0, x=w427) -> (x << y=w430:u32[])
          n177 = Logical Shift(y=i16 8, x=w427) -> (x << y=w429:u32[])
          n178 = Logical Shift(y=i16 16, x=w427) -> (x << y=w428:u32[])
          n179 = Compound Arithmetic op=ADD(w430, w429, w428) -> (w431:u32[])
          n180 = Rotate 1D Array(1:w431, 2:w435) -> (0:w425:u32[])
        }
        frame "YELLOW, BLINK" {
          n181 = local read "array YELLOW"() -> (w437:u32[])
          n182 = local read "array BLACK"() -> (w436:u32[])
        }
        frame "YELLOW, BUMPER" {
          n183 = local read "array YELLOW"() -> (w440:u32[])
          n184 = local read "array BLACK"() -> (w439:u32[])
        }
        frame "YELLOW, SCAN" {
          n185 = local read "array YELLOW"() -> (w443:u32[])
          n186 = local read "array BLACK"() -> (w442:u32[])
        }
        frame "YELLOW, SOLID" {
          n187 = local read "array YELLOW"() -> (w446:u32[])
          n188 = local read "array BLACK"() -> (w445:u32[])
        }
      }
      n189 = case shown="\"SCAN FAST\"" w47 {
        tunnel: w51 -> [w53 w59 w71 w83 w94 w109 w113 w123 w140 w161 w169 w175]
        tunnel: [w53 w56 w68 w80 w91 w106 w113 w127 w144 w163 w167 w175] -> w50
        tunnel: w49 -> [_ w55 w67 w79 w90 w102 _ w122 w139 w160 w168 _]
        tunnel: [w52 w54 w66 w78 w88 w104 w112 w114 w131 w148 w165 w174] -> w48
        frame "SOLID", Default {
          n190 = local read "DesiredLoopTime_MS"() -> (w52:dbl)
        }
        frame "BUMPER" {
          n191 = local read "slider length"() -> (w57:i8)
          n192 = local read "SCAN rotation"() -> (w62:dbl)
          n193 = Array Subset(array=w59, index=0, length=w57) -> (w60:u32[])
          n194 = To Long Integer(number=w62) -> (32bit integer=w61:i32)
          n195 = call "overlay LED colors.vi"("BASE ARRAY"=w55, "OVERLAY"=w60) -> ("BLENDED ARRAY"=w63:u32[])  [unwired: 9 in]
          n196 = Rotate 1D Array(1:w63, 2:w61) -> (0:w56:u32[])
          n197 = local read "LOOP - BUMPER (ms)"() -> (w54:dbl)
        }
        frame "BUMPER FAST" {
          n198 = local read "slider length"() -> (w69:i8)
          n199 = local read "SCAN rotation"() -> (w74:dbl)
          n200 = Array Subset(array=w71, index=0, length=w69) -> (w72:u32[])
          n201 = Scale By Power Of 2(n=i16 1, x=w74) -> (x*2^n=w65:dbl)
          n202 = To Long Integer(number=w65) -> (32bit integer=w73:i32)
          n203 = call "overlay LED colors.vi"("BASE ARRAY"=w67, "OVERLAY"=w72) -> ("BLENDED ARRAY"=w75:u32[])  [unwired: 9 in]
          n204 = Rotate 1D Array(1:w75, 2:w73) -> (0:w68:u32[])
          n205 = local read "LOOP - BUMPER (ms)"() -> (w66:dbl)
        }
        frame "FIBONACCI" {
          n206 = local read "slider length"() -> (w81:i8)
          n207 = local read "SCAN rotation"() -> (w86:dbl)
          n208 = Array Subset(array=w83, index=0, length=w81) -> (w84:u32[])
          n209 = Scale By Power Of 2(n=i16 1, x=w86) -> (x*2^n=w77:dbl)
          n210 = To Long Integer(number=w77) -> (32bit integer=w85:i32)
          n211 = call "overlay LED colors.vi"("BASE ARRAY"=w79, "OVERLAY"=w84) -> ("BLENDED ARRAY"=w87:u32[])  [unwired: 9 in]
          n212 = Rotate 1D Array(1:w87, 2:w85) -> (0:w80:u32[])
          n213 = local read "LOOP - BUMPER (ms)"() -> (w78:dbl)
        }
        frame "SCAN" {
          n214 = local read "slider length"() -> (w92:i8)
          n215 = local read "FORWARD INDEX"() -> (w89:i32)
          n216 = Array Subset(array=w94, index=0, length=w92) -> (w95:u32[])
          n217 = call "overlay LED colors.vi"("BASE ARRAY"=w90, "OVERLAY"=w95) -> ("BLENDED ARRAY"=w96:u32[])  [unwired: 9 in]
          n218 = Rotate 1D Array(1:w96, 2:w89) -> (0:w91:u32[])
          n219 = local read "LOOP - SCAN (ms)"() -> (w88:dbl)
        }
        frame "SCAN FAST" {
          n220 = Array Size(array=w102) -> (size(s)=w100:i32)
          n221 = local read "slider length"() -> (w107:i8)
          n222 = Divide(x=w100, y=2) -> (x/y=w101:dbl)
          n223 = Array Subset(array=w109, index=0, length=w107) -> (w110:u32[])
          n224 = call "overlay LED colors.vi"("BASE ARRAY"=w102, "OVERLAY"=w110) -> ("BLENDED ARRAY"=w111:u32[])  [unwired: 9 in]
          n225 = local read "FORWARD INDEX"() -> (w105:i32)
          n226 = Array Subset(array=w111, index=0, length=w101) -> (w97:u32[])
          n227 = local read "LOOP - SCAN (ms)"() -> (w104:dbl)
          n228 = Build Array (concatenate)(w97, w97) -> (w98:u32[])
          n229 = Rotate 1D Array(1:w98, 2:w105) -> (0:w106:u32[])
        }
        frame "WAVE" {
          n230 = local read "LOOP - WAVE (ms)"() -> (w112:dbl)
        }
        frame "EXPAND" {
          n231 = local read "#LEDs"() -> (w118:T2)
          n232 = local read "HEARTBEAT"() -> (w115:i32)
          n233 = Divide(x=w118, y=u16 2) -> (x/y=w120:dbl)
          n234 = Quotient & Remainder(x=w115, y=w120) -> (x-y*floor(x/y)=w119:dbl)  [unwired: 1 out]
          n235 = To Unsigned Word Integer(number=w120) -> (unsigned 16bit integer=w117:u16)
          n236 = To Unsigned Word Integer(number=w119) -> (unsigned 16bit integer=w116:u16)
          n237 = Array Subset(array=w122, index=0, length=w117) -> (w124:u32[])
          n238 = Array Subset(array=w123, index=0, length=w116) -> (w130:u32[])
          n239 = call "overlay LED colors.vi"("BASE ARRAY"=w124, "OVERLAY"=w130) -> ("BLENDED ARRAY"=w126:u32[])  [unwired: 9 in]
          n240 = local read "LOOP - SCAN (ms)"() -> (w114:dbl)
          n241 = Reverse 1D Array(array=w126) -> (reversed array=w128:u32[])
          n242 = Build Array (concatenate)(w128, w126) -> (w127:u32[])
        }
        frame "EX-CON" {
          n243 = local read "#LEDs"() -> (w135:T2)
          n244 = local read "SINE 0-1"() -> (w132:dbl)
          n245 = Divide(x=w135, y=u16 2) -> (x/y=w137:dbl)
          n246 = Multiply(x=w132, y=w137) -> (x*y=w136:dbl)
          n247 = To Unsigned Word Integer(number=w137) -> (unsigned 16bit integer=w134:u16)
          n248 = To Unsigned Word Integer(number=w136) -> (unsigned 16bit integer=w133:u16)
          n249 = Array Subset(array=w139, index=0, length=w134) -> (w141:u32[])
          n250 = Array Subset(array=w140, index=0, length=w133) -> (w147:u32[])
          n251 = call "overlay LED colors.vi"("BASE ARRAY"=w141, "OVERLAY"=w147) -> ("BLENDED ARRAY"=w143:u32[])  [unwired: 9 in]
          n252 = local read "LOOP - SCAN (ms)"() -> (w131:dbl)
          n253 = Reverse 1D Array(array=w143) -> (reversed array=w145:u32[])
          n254 = Build Array (concatenate)(w145, w143) -> (w144:u32[])
        }
        frame "CROSS" {
          n255 = local read "slider length"() -> (w159:i8)
          n256 = local read "SCAN rotation"() -> (w153:dbl)
          n257 = local read "array BLACK"() -> (w156:u32[])
          n258 = Array Subset(array=w161, index=0, length=w159) -> (w157:u32[])
          n259 = Array Subset(array=w160, index=0, length=w159) -> (w158:u32[])
          n260 = call "overlay LED colors.vi"("BASE ARRAY"=w156, "OVERLAY"=w157) -> ("BLENDED ARRAY"=w155:u32[])  [unwired: 9 in]
          n261 = call "overlay LED colors.vi"("BASE ARRAY"=w156, "OVERLAY"=w158) -> ("BLENDED ARRAY"=w154:u32[])  [unwired: 9 in]
          n262 = To Long Integer(number=w153) -> (32bit integer=w152:i32)
          n263 = Rotate 1D Array(1:w155, 2:w152) -> (0:w151:u32[])
          n264 = Rotate 1D Array(1:w154, 2:w152) -> (0:w150:u32[])
          n265 = Reverse 1D Array(array=w150) -> (reversed array=w149:u32[])
          n266 = local read "LOOP - SCAN (ms)"() -> (w148:dbl)
          n267 = Add(x=w151, y=w149) -> (x+y=w163:u32[])
        }
        frame "BLINK" {
          n268 = local read "HEARTBEAT"() -> (w166:i32)
          n269 = Quotient & Remainder(x=w166, y=10) -> (x-y*floor(x/y)=w172:i32)  [unwired: 1 out]
          n270 = Greater Or Equal?(x=w172, y=5) -> (x >= y?=w170:bool)
          n271 = Select(t=w169, s=w170, f=w168) -> (s? t:f=w167:u32[])
          n272 = local read "LOOP - BLINK (ms)"() -> (w165:dbl)
        }
        frame "PULSE" {
          n273 = local read "DesiredLoopTime_MS"() -> (w174:dbl)
        }
      }
    }
    n274 = in-place {
      in-place-border: w42 -> [w449]
      # "VALUE of 0 @ CLOCK = 0\nto 1 @ CLOCK = #LEDs"
      n275 = local read "#LEDs"() -> (w453:T2)
      n276 = Quotient & Remainder(x=w449, y=w453) -> (x-y*floor(x/y)=w459:i32)  [unwired: 1 out]
      "FORWARD INDEX" <- w459
      n277 = Decrement(x=w453) -> (x-1=w462:T2)
      n278 = Divide(x=6.283185307179586, y=w453) -> (x/y=w460:dbl)
      n279 = Subtract(x=w453, y="slider length") -> (x-y=w451:T2)
      n280 = Subtract(x=w462, y=w459) -> (x-y=→"REVERSE INDEX":i32)
      n281 = Multiply(x=w459, y=w460) -> (x*y=w458:dbl)
      n282 = Subtract(x=w462, y="slider length") -> (x-y=→"REVERSE BUMP":T2)
      n283 = Initialize Array(u32 0 ("Color2"), "slider length") -> (→"SLIDER BLACK":u32[])
      n284 = Initialize Array(u32 16448250 ("Color2"), "slider length") -> (→"SLIDER WHITE":u32[])
      n285 = Cosine(x=w458) -> (cos(x)=w457:dbl)
      n286 = Add(x=w457, y=1.0) -> (x+y=w455:dbl)
      n287 = Divide(x=w455, y=2.0) -> (x/y=w448:dbl)
      "SINE 0-1" <- w448
      n288 = Multiply(x=w451, y=w448) -> (x*y=→"SCAN rotation":dbl)
      "HEARTBEAT" <- w449
    }
    n289 = in-place {
      in-place-border: w40 -> [w469]
      w471 = 10.0  # MaxDeviation_MS
      n290 = in-place {
      }
      n291 = call <vilib>:"Time_WaitAdjust.vi"("MaxAdjustment_MS"=w471, "DesiredLoopTime_MS"=w469) -> ("AdjustedWaitTime_MS"=w470:u32)  [unwired: 8 in, 1 out]
      "AdjustedWaitTime_MS" <- w470
      n292 = Wait (ms)(milliseconds to wait=w470) -> ()  [unwired: 1 out]
    }
    n293 = in-place {
      in-place-border: w41 -> [w472]
      n294 = local read "TESTING?"() -> (w473:bool)
      n295 = case shown="False" w473 {
        tunnel: w472 -> [w474 w476]
        frame False {
          n296 = call <vilib>:"WPI_LED_Write.vi"("Color Array"=w474) -> ()  [unwired: 10 in, 1 out]
        }
        frame True {
          n297 = local read "#LEDs"() -> (w478:T2)
          n298 = Divide(x=w478, y=T2 2) -> (x/y=w475:dbl)
          n299 = Split 1D Array(array=w476, index=w475) -> (first subarray=→"LED WRITE 2":u32[], second subarray=→"LED WRITE 3":u32[])
        }
      }
      "LED WRITE" <- w472
    }
  }
  n300 = global read "Global INIT.vi" "LED init"() -> (w2:T4)
  n301 = in-place {
    w488 = 0.0 ("element")
    n302 = Increment(x=w488) -> (x+1=w487:dbl)
    n303 = local read "#LEDs"() -> (w484:T2)
    n304 = Build Array(w487) -> (w489:dbl[])
    n305 = while {
      shift-right: [w494] -> _
      shift-left: w487 -> [w496]
      shift-left: w488 -> [w495]
      shift-right: [w497] -> w483
      shift-left: w489 -> [w498]
      shift-right: [w491] -> w485
      shift-left: 0.0 -> [w493]
      tunnel: w484 -> [w490]
      stop <- w492 stop-if-true
      n306 = Add(x=w496, y=w495) -> (x+y=w494:dbl)
      n307 = Add(x=w494, y=w493) -> (x+y=w491:dbl)
      n308 = Build Array (concatenate)(w498, w494) -> (w497:dbl[])
      n309 = Greater Or Equal?(x=w491, y=w490) -> (x >= y?=w492:bool)
    }
    "FIBONACCI array" <- w483
    "Numeric" <- w485
    n310 = Decimate 1D Array(w483) -> (→"decimated array":dbl[], →"decimated array 2":dbl[])
  }
  n311 = Unbundle By Name(w2) -> ("#LEDS"=w1:T2)
  "#LEDs" <- w1
  n312 = Scale By Power Of 2(n=i16 30, x=1.0) -> (x*2^n=w19:dbl)
  n313 = Initialize Array("ORANGE", w1) -> (→"array ORANGE":u32[])
  n314 = Initialize Array("YELLOW", w1) -> (→"array YELLOW":u32[])
  n315 = Initialize Array("Color1", w1) -> (→"array COLOR1":u32[])
  n316 = Initialize Array("PINK", w1) -> (→"array PINK":u32[])
  n317 = Initialize Array("Color2", w1) -> (→"array COLOR2":u32[])
  n318 = Initialize Array("Dk BLUE", w1) -> (→"array DK BLUE":u32[])
  n319 = Initialize Array(w19, w1) -> (→"array EMPTY":dbl[])
  n320 = Initialize Array("FUSCIA", w1) -> (→"array FUSCIA":u32[])
  n321 = Initialize Array("VIOLET", w1) -> (→"array VIOLET":u32[])
  n322 = Initialize Array("GREEN", w1) -> (→"array GREEN":u32[])
  n323 = Initialize Array(u32 61414 ("Color2"), w1) -> (→"array AQUA":u32[])
  n324 = Initialize Array(u32 220 ("Color2"), w1) -> (→"array BLUE":u32[])
  n325 = Initialize Array(u32 16711680 ("Color2"), w1) -> (→"array RED":u32[])
  n326 = Initialize Array(u32 16448250 ("Color2"), w1) -> (→"array WHITE":u32[])
  n327 = Initialize Array(u32 0 ("Color2"), w1) -> (→"array BLACK":u32[])
  n328 = Divide(x=6.283185307179586, y=w1) -> (x/y=w13:dbl)
  n329 = for {
    N: w1 -> [_]
    tunnel: w13 -> [w502]
    tunnel: [w514] -> w12 mode=indexing
    tunnel: [w500] -> w11 mode=indexing
    i -> [w503]
    # "0..255"
    # "start at lowest value"
    # "0..1"
    # "0..2"
    n330 = Multiply(x=w502, y=w503) -> (x*y=w519:dbl)
    n331 = Compound Arithmetic op=MULTIPLY(w503, w502, 2.0 ("value")) -> (w509:dbl)
    n332 = Subtract(x=w519, y=1.5707963267948966) -> (x-y=w518:dbl)
    n333 = Subtract(x=w509, y=1.5707963267948966) -> (x-y=w508:dbl)
    n334 = Sine(x=w518) -> (sin(x)=w523:dbl)
    n335 = Sine(x=w508) -> (sin(x)=w513:dbl)
    n336 = Add(x=w523, y=1.0) -> (x+y=w521:dbl)
    n337 = Add(x=w513, y=1.0) -> (x+y=w511:dbl)
    n338 = Divide(x=w511, y=2.0) -> (x/y=w506:dbl)
    n339 = Divide(x=w521, y=2.0) -> (x/y=w499:dbl)
    n340 = Multiply(x=w506, y=255.0) -> (x*y=w505:dbl)
    n341 = Multiply(x=w499, y=255.0) -> (x*y=w516:dbl)
    n342 = To Unsigned Long Integer(number=w516) -> (unsigned 32bit integer=w514:u32)
    n343 = To Unsigned Long Integer(number=w505) -> (unsigned 32bit integer=w500:u32)
  }
  "SINE WAVE" <- w12
  "SINE WAVE 1/2" <- w11
